vi "sub_data.vi"(7 "cmd":enum16{"ini", "write", "read"}(ring), 8 "error in (no error)":errorcluster caption="에러 입력(에러 없음)", 11 "data in":T1) -> (0 "error out":errorcluster caption="에러 출력", 3 "data out":T1)   [LabVIEW 2016]
uses:
  ctl/data.ctl
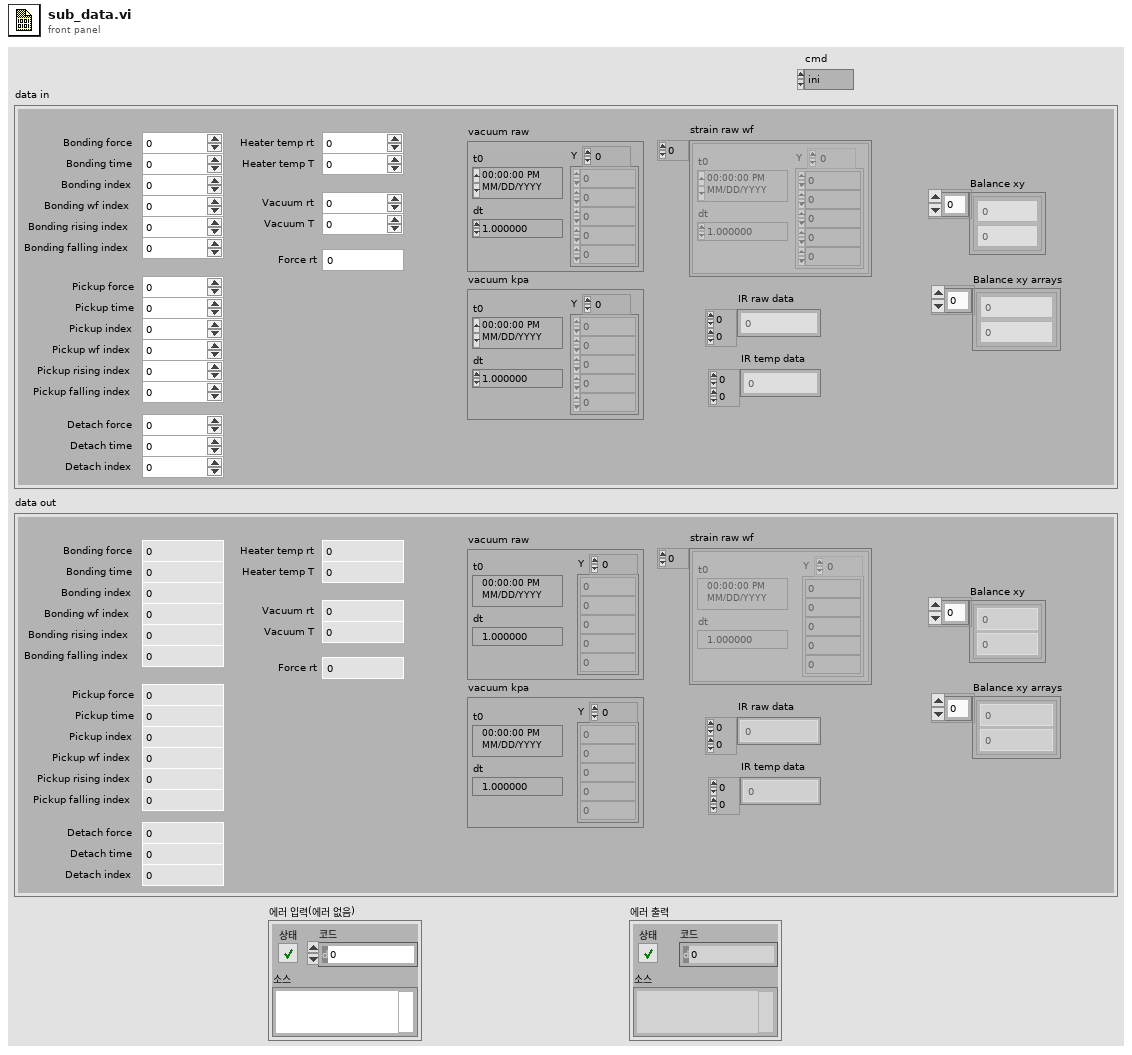
[diagram p1: front panel]
types:
  T1 = typedef "data.ctl" = cluster{"Bonding force":dbl, "Bonding time":dbl, "Bonding index":dbl, "Pickup force":dbl, "Pickup time":dbl, "Pickup index":dbl, "Detach force":dbl, "Detach time":dbl, "Detach index":dbl, "Heater temp rt":dbl, "Vacuum rt":dbl, "IR raw data":i16[][], "IR temp data":dbl[][], "vacuum raw wf":waveform(dbl), "vacuum kpa wf":waveform(dbl), "strain raw wf":waveform(dbl)[], "Force rt":dbl, "Vacuum T":dbl, "Heater temp T":dbl, "Balance xy arrays":cluster{dbl, dbl}[], "Balance xy":cluster{dbl, dbl}[], "Bonding wf index":dbl, "Pickup wf index":dbl, "Bonding rising index":dbl, "Bonding falling index":dbl, "Pickup rising index":dbl, "Pickup falling index":dbl}
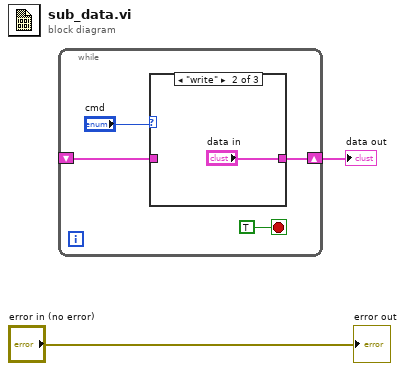
[diagram p0: block diagram]
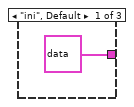
[diagram p2: hidden frame]
diagram:
  n1 = while {
    shift-right: [w4] -> w2
    shift-left: _ -> [w3]
    stop <- TRUE stop-if-true
    n2 = case shown="\"write\"" "cmd" {
      tunnel: [T1 {"Bonding force"=0.0, "Bonding time"=0.0, "Bonding index"=0.0, "Pickup force"=0.0, "Pickup time"=0.0, "Pickup index"=0.0, "Detach force"=0.0, "Detach time"=0.0, "Detach index"=0.0, "Heater temp rt"=0.0, "Vacuum rt"=0.0, "IR raw data"=[], "IR temp data"=[], "vacuum raw wf"={"t0"=timestamp(0 s since 1904-01-01), "dt"=1.0, "Y"=[]}, "vacuum kpa wf"={"t0"=timestamp(0 s since 1904-01-01), "dt"=1.0, "Y"=[]}, "strain raw wf"=[], "Force rt"=0.0, "Vacuum T"=0.0, "Heater temp T"=0.0, "Balance xy arrays"=[], "Balance xy"=[], "Bonding wf index"=0.0, "Pickup wf index"=0.0, "Bonding rising index"=0.0, "Bonding falling index"=0.0, "Pickup rising index"=0.0, "Pickup falling index"=0.0} ("data out 2") "data in" w9] -> w4
      tunnel: w3 -> [_ _ w9]
      frame "ini", Default {
      }
      frame "write" {
      }
      frame "read" {
      }
    }
  }
  "data out" <- w2
  "error out" <- "error in (no error)"
